vi "Read sunProximity.vi"(8 "error in (no error)":errorcluster, 11 "Limits in":refnum<class "Limits.lvclass">) -> (0 "error out":errorcluster, 2 "SunMoonStatus.lvclass":refnum<class "SunMoonStatus.lvclass">, 3 "Limits out":refnum<class "Limits.lvclass">)   [LabVIEW 2014, in "TCSDataDefinitions.lvlib" / "TCSPublicStatus.lvlib" / "Limits.lvlib" / "Limits.lvclass"]
uses:
  Limits.lvclass
  SunMoonStatus/SunMoonStatus.lvclass
  Limits.lvclass/Limits.ctl
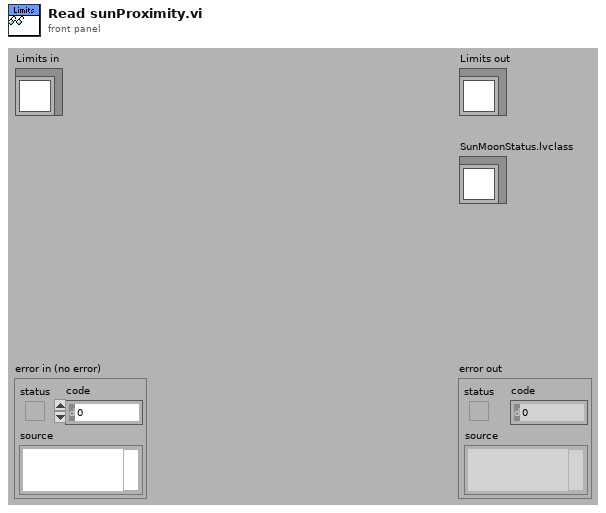
[diagram p1: front panel]
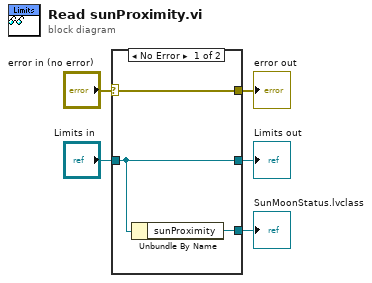
[diagram p0: block diagram]
diagram:
  n1 = case shown="No Error" "error in (no error)" {
    selector: "error in (no error)" -> [w8 w9]
    tunnel: [w8 w9] -> w4
    tunnel: [w7 w10] -> w2
    tunnel: "Limits in" -> [w7 w10]
    tunnel: [w6 _] -> w1
    frame No Error {
      n2 = Unbundle By Name(w7) -> ("sunProximity"=w6:refnum<class "SunMoonStatus.lvclass">)
    }
    frame Error {
    }
  }
  "error out" <- w4
  "Limits out" <- w2
  "SunMoonStatus.lvclass" <- w1
